vi "Set - SigMath User Ctrl Refs.vi"(0 "reference in":refnum<class "SigMath.lvclass">, 5 "error in (no error)":errorcluster, 7 "User CTRL Refs":T1) -> (14 "reference out":refnum<class "SigMath.lvclass">, 19 "error out":errorcluster)   [LabVIEW 2020, in "SigMath.lvclass"]
uses:
  SigMath.lvclass
  protected/SigMath User CTRL Refs.ctl
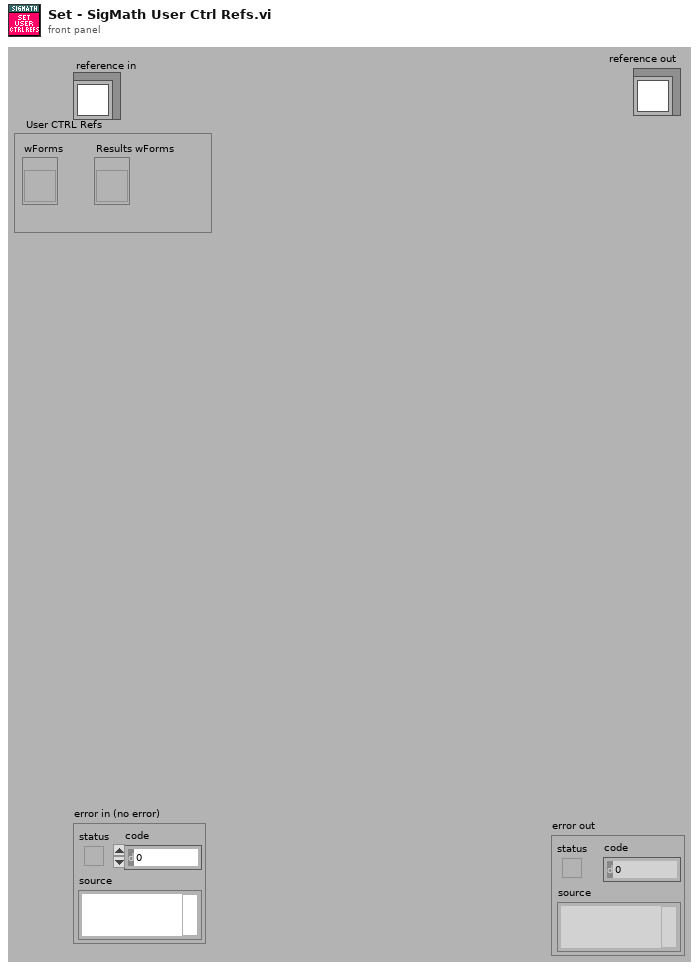
[diagram p1: front panel]
types:
  T1 = typedef "SigMath.lvclass/SigMath User CTRL Refs.ctl" = cluster{"wForms":refnum<vi>, "Results wForms":refnum<vi>}
  T2 = typedef "SigMath.lvclass/ObjectAttributesRef.ctl" = refnum<data-value>
  T3 = typedef "SigMath.lvclass/ObjectAttributes.ctl" = cluster{"SigMath Data":T4, "User CTRL Refs":T1}
  T4 = typedef "SigMath.lvclass/SigMath Data.ctl" = cluster{"New Time Data Obj?":bool, "GSwFormDSP":refnum<class "GSwFormDSP.lvclass">}
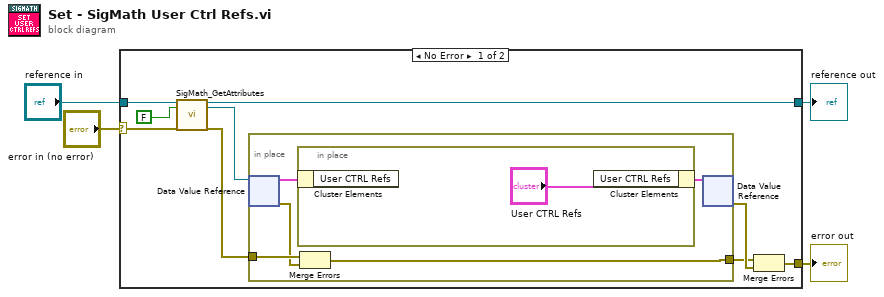
[diagram p0: block diagram]
diagram:
  n1 = case shown="No Error" "error in (no error)" {
    selector: "error in (no error)" -> [w8 w21]
    tunnel: [w13 w21] -> w3
    tunnel: [w7 w20] -> w1
    tunnel: "reference in" -> [w10 w20]
    frame No Error {
      n2 = call "SigMath_GetAttributes.vi"("reference in"=w10, "return data? (T)"=FALSE, "error in (no error)"=w8) -> ("reference out"=w7:refnum<class "SigMath.lvclass">, "attributes ref"=w6:T2, "error out"=w5:errorcluster)  [unwired: 13 in, 1 out]
      n3 = in-place {
        in-place-border: [w14] -> w11
        in-place-border: w5 -> [w16]
        n4 = in-place-dvr #1(w6) -> (w17:T3, w15:errorcluster)
        n5 = in-place {
          n6 = in-place-cluster #2(w17) -> ()  [unwired: 1 out]
          n7 = in-place-cluster #2("User CTRL Refs"="User CTRL Refs") -> (w18:T3)
        }
        n8 = Merge Errors(w16, w15) -> (w14:errorcluster)
        n9 = in-place-dvr #1(w18) -> (w12:errorcluster)  [unwired: 1 out]
      }
      n10 = Merge Errors(w11, w12) -> (w13:errorcluster)
    }
    frame Error {
    }
  }
  "error out" <- w3
  "reference out" <- w1
